vi "Sub_ConvertTemperatureMatrixIntoColorMatrix.vi"(2 "Lower temperature bound":dbl, 3 "Upper temperature bound":dbl, 4 "Input temperature matrix":T1) -> (0 "Output color boxes":u32[][](array[colorbox]), 1 "Output color codes":u32[][](array[numeric]) format="%x")   [LabVIEW 2018]
uses:
  <vilib>/Analysis/Matrix/Datatypes/RealMatrix.ctl
  <vilib>/Analysis/Matrix/NI_Matrix.lvlib
panel:
  # "Inputs:"
  # "Outputs:"
  # "Required:"
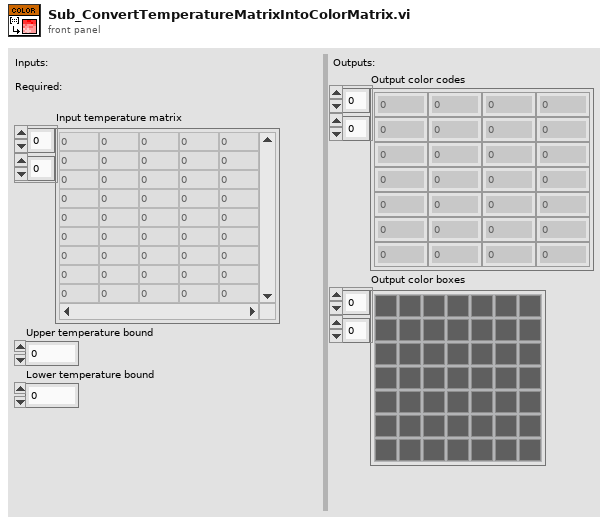
[diagram p1: front panel]
types:
  T1 = typedef "NI_Matrix.lvlib/RealMatrix.ctl" = dbl[][]
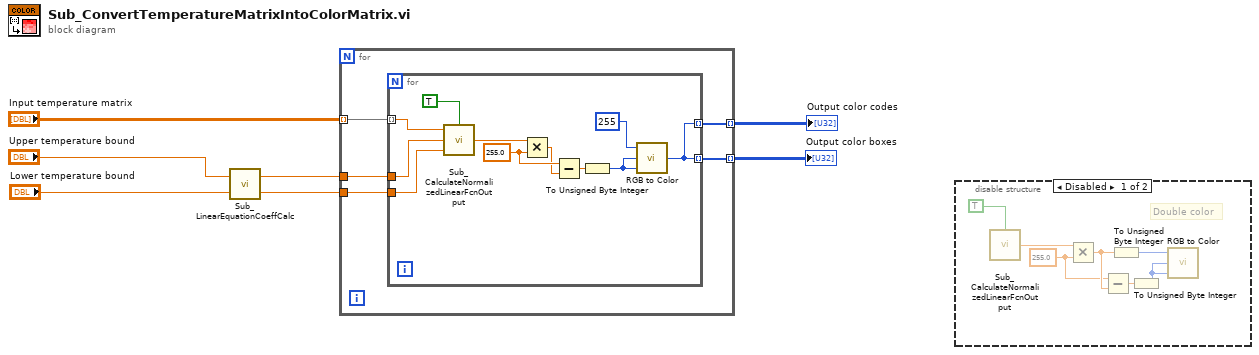
[diagram p0: block diagram]
diagram:
  n1 = call "Sub_LinearEquationCoeffCalc.vi"("Lower bound"="Lower temperature bound", "Upper bound"="Upper temperature bound") -> ("B"=w4:dbl, "A"=w5:dbl)
  n2 = for {
    tunnel: w5 -> [w11]
    tunnel: w4 -> [w10]
    tunnel: "Input temperature matrix" -> [w12] mode=indexing
    tunnel: [w9] -> w2 mode=indexing
    tunnel: [w8] -> w1 mode=indexing
    n3 = for {
      tunnel: w12 -> [w22] mode=indexing
      tunnel: w11 -> [w21]
      tunnel: w10 -> [w20]
      tunnel: [w19] -> w9 mode=indexing
      tunnel: [w19] -> w8 mode=indexing
      w17 = 255.0 ("y")
      n4 = call "Sub_CalculateNormalizedLinearFcnOutput.vi"("Saturate to 0-1 ?"=TRUE, "B coefficient"=w20, "A coefficient"=w21, "Value"=w22) -> ("Normalized value"=w18:dbl)
      n5 = Multiply(x=w18, y=w17) -> (x*y=w16:dbl)
      n6 = Subtract(x=w17, y=w16) -> (x-y=w15:dbl)
      n7 = To Unsigned Byte Integer(number=w15) -> (unsigned 8bit integer=w14:u8)
      n8 = call <vilib>:"RGB to Color.vi"("B"=w14, "G"=w14, "R"=u8 255 ("G")) -> ("Color"=w19:u32)
    }
  }
  "Output color boxes" <- w2
  "Output color codes" <- w1
  n9 = disable-structure shown="Disabled" {
    frame Disabled {
      w27 = 255.0 ("y")
      # "Double color"
      n10 = call "Sub_CalculateNormalizedLinearFcnOutput.vi"("Saturate to 0-1 ?"=TRUE) -> ("Normalized value"=w25:dbl)  [unwired: 3 in]
      n11 = Multiply(x=w25, y=w27) -> (x*y=w28:dbl)
      n12 = Subtract(x=w27, y=w28) -> (x-y=w29:dbl)
      n13 = To Unsigned Byte Integer(number=w28) -> (unsigned 8bit integer=w26:u8)
      n14 = To Unsigned Byte Integer(number=w29) -> (unsigned 8bit integer=w30:u8)
      n15 = call <vilib>:"RGB to Color.vi"("B"=w30, "G"=w30, "R"=w26) -> ()  [unwired: 1 out]
    }
    frame Enabled {
    }
  }
